vi "CalcThetaFromX.vi"(11 "X":dbl) -> (3 "Numeric":dbl)   [LabVIEW 2018]
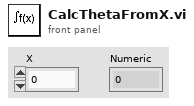
[diagram p1: front panel]
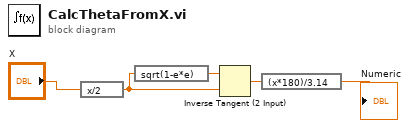
[diagram p0: block diagram]
diagram:
  n1 = expression code="x/2"("X") -> (w2:dbl)
  n2 = expression code="sqrt(1-e*e)"(w2) -> (w3:dbl)
  n3 = Inverse Tangent (2 Input)(1:w2, 2:w3) -> (0:w4:dbl)
  n4 = expression code="(x*180)/3.14"(w4) -> (→"Numeric":dbl)
